vi "Set PanelVIRefs.vi"(8 "error in (no error)":errorcluster caption="错误输入（无错误）", 11 "PanelRootNode 输入":refnum<class "PanelRootNode.lvclass"> caption="DNL_LabVIEW Object in") -> (0 "error out":errorcluster caption="错误输出", 1 "VerticalPanel":refnum<vi>, 2 "HorizontalPanel":refnum<vi>, 3 "PanelRootNode 输出":refnum<class "PanelRootNode.lvclass"> caption="DNL_LabVIEW Object out")   [LabVIEW 2016, in "PanelRootNode.lvclass"]
uses:
  PanelRootNode.lvclass
  PanelDataNode/PanelDataNode.lvclass
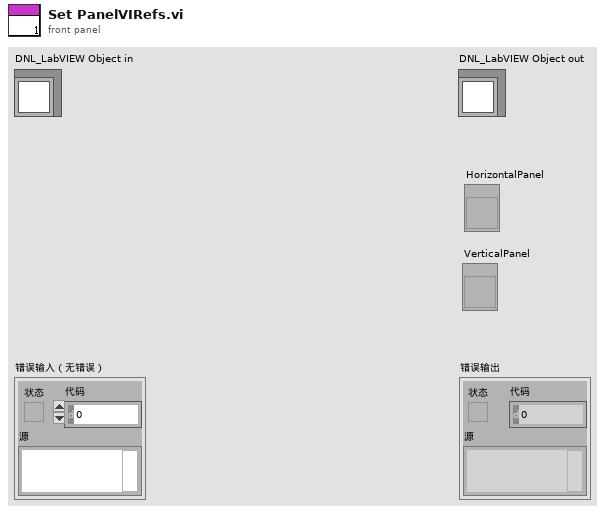
[diagram p1: front panel]
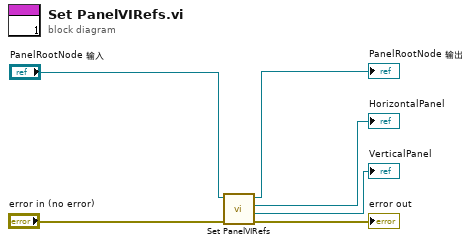
[diagram p0: block diagram]
diagram:
  n1 = call-parent "Set PanelVIRefs.vi"("error in (no error)"="error in (no error)", "PanelDataNode 输入"="PanelRootNode 输入") -> ("error out"=→"error out":errorcluster, "VerticalPanel"=→"VerticalPanel":refnum<vi>, "HorizontalPanel"=→"HorizontalPanel":refnum<vi>, "PanelDataNode 输出"=→"PanelRootNode 输出":refnum<class "PanelRootNode.lvclass">)  [unwired: 6 in]
